vi "MoveHWP primitive v2.vi"(6 "tolerance":sgl, 7 "StopCtrl":bool, 8 "error in (no error)":errorcluster, 9 "DesiredAngle":sgl, 10 "HomeTheStage":bool, 11 "Automation Refnum in":refnum<k7>) -> (0 "error out":errorcluster, 1 "running error out":errorcluster, 2 "GetPosition_Position":sgl, 3 "GetStatusBits_Bits continual":i32 format="%b", 5 "CurrentAngle":sgl)   [LabVIEW 2013]
uses:
  <vilib>/Analysis/1siggen.llb/Ramp Pattern by Delta.vi
  <vilib>/Analysis/NI_AALBase.lvlib
panel:
  out "Array":sgl[](array[numeric])
  out "XY Graph":T1(graph)
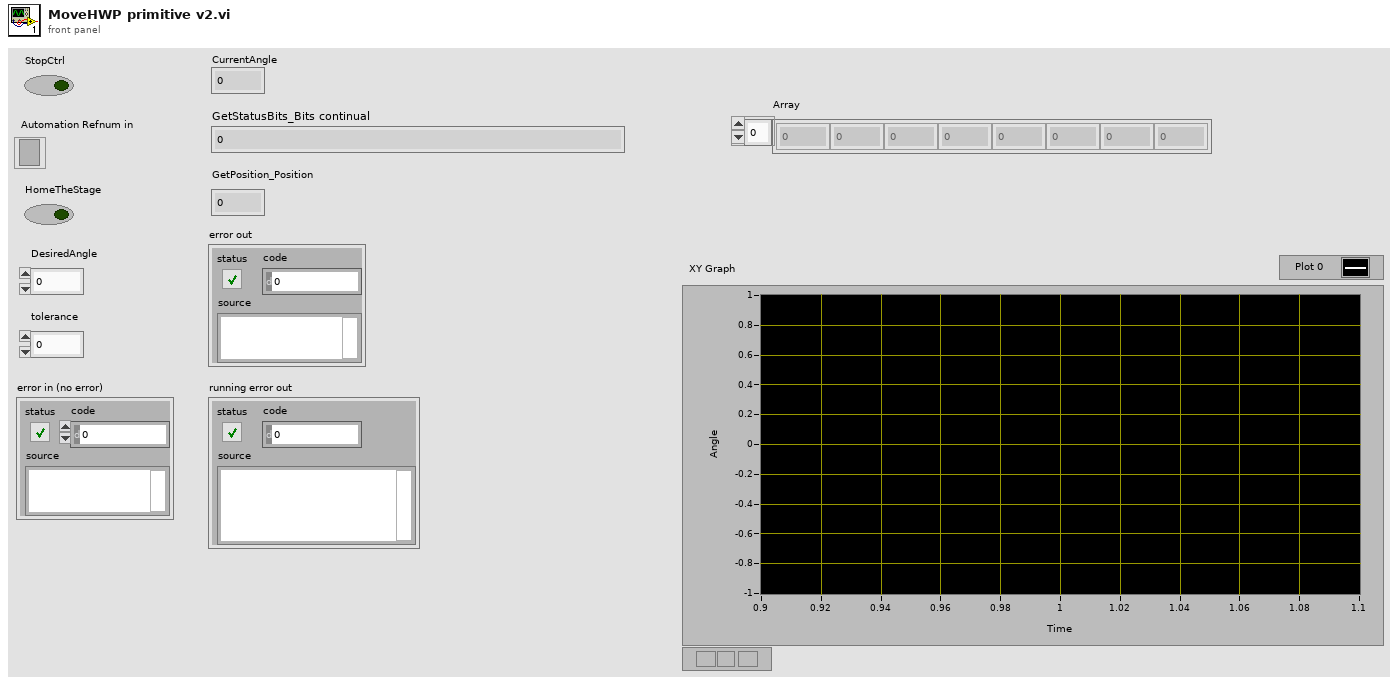
[diagram p1: front panel]
types:
  T1 = cluster{"Ramp Pattern":dbl[], "Array of Continuous Angles":dbl[]}
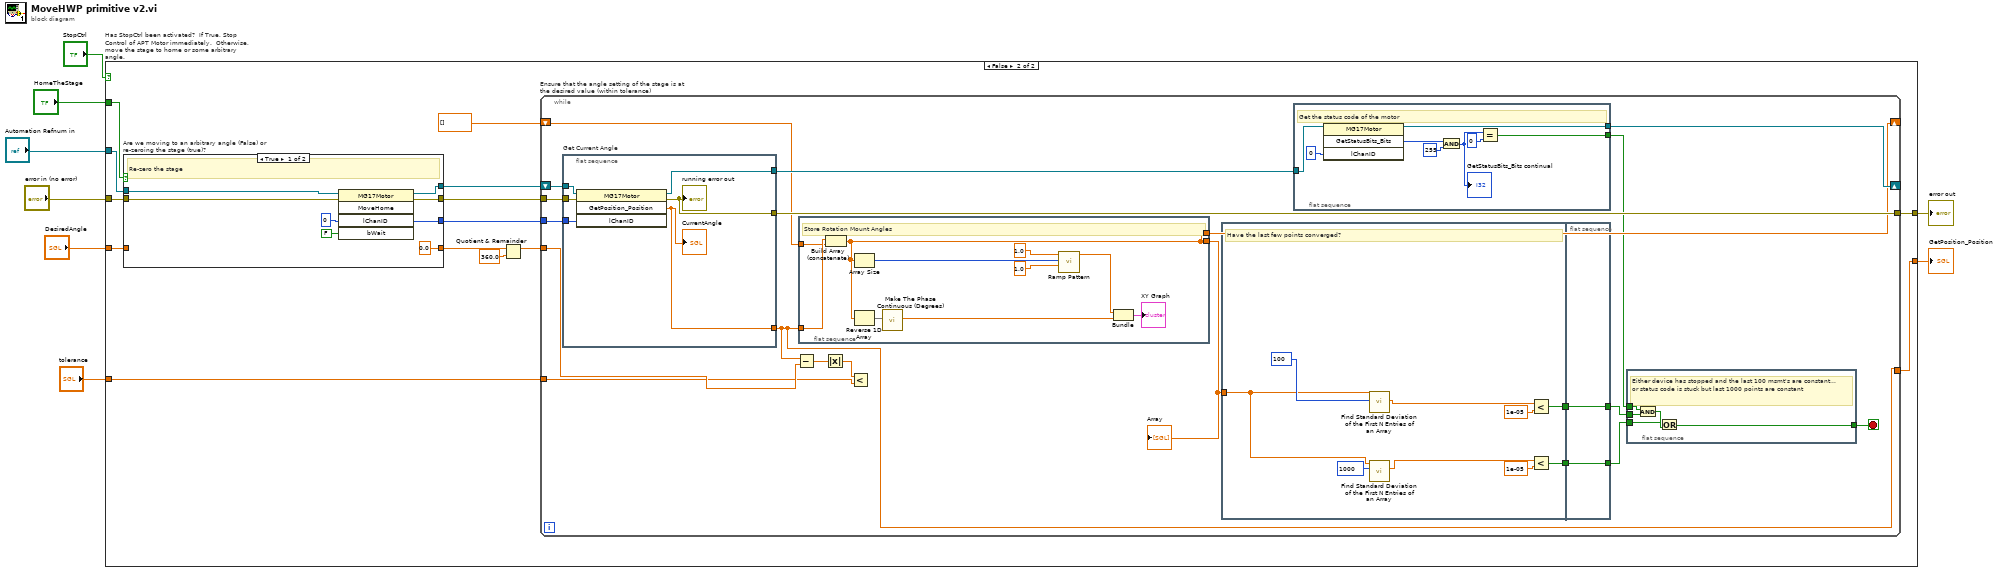
[diagram p0: block diagram]
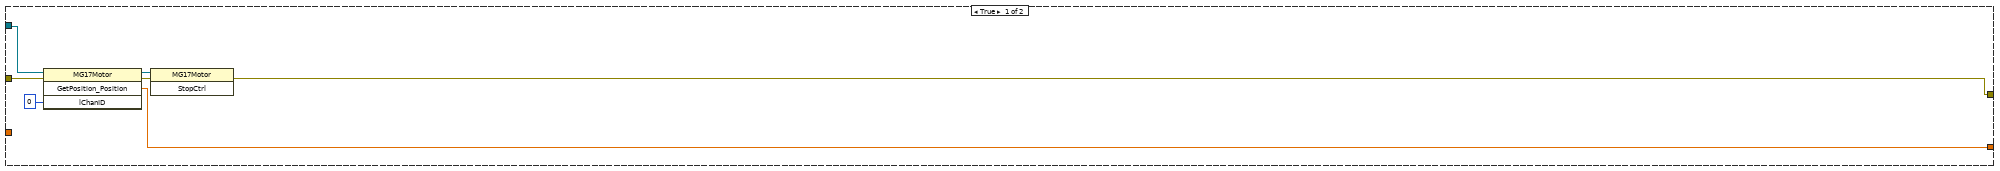
[diagram p2: hidden frame]
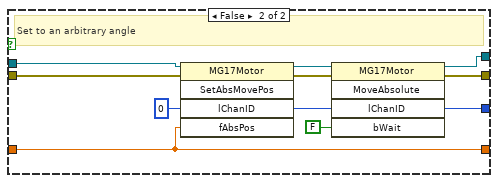
[diagram p3: hidden frame]
diagram:
  n1 = case "Has StopCtrl been activated?  If True, Stop Control of APT Motor immediately.  Otherwise, move the stage to home or some arbitrary angle." shown="False" "StopCtrl" {
    tunnel: "Automation Refnum in" -> [w15 w29]
    tunnel: "error in (no error)" -> [w14 w28]
    tunnel: [w10 w22] -> w3
    tunnel: [w9 w23] -> w2
    tunnel: "HomeTheStage" -> [_ w20]
    tunnel: "DesiredAngle" -> [_ w19]
    tunnel: "tolerance" -> [_ w18]
    frame True {
      n2 = invoke class="MG17Motor" method="GetPosition_Position"(reference=w15, error in=w14, "lChanID"=0) -> (reference out=w12:refnum<k7>, error out=w11:errorcluster, "GetPosition_Position"=w9:sgl)  [unwired: 1 in, 1 out]
      n3 = invoke class="MG17Motor" method="StopCtrl"(reference=w12, error in=w11) -> (error out=w10:errorcluster)  [unwired: 1 in, 2 out]
    }
    frame False {
      n4 = case "Are we moving to an arbitrary angle (False) or re-zeroing the stage (true)?" shown="True" w20 {
        tunnel: w29 -> [w95 w103]
        tunnel: w28 -> [w94 w102]
        tunnel: [w93 w101] -> w27
        tunnel: [sgl 0.0 ("Angle") w98] -> w26
        tunnel: [w91 w99] -> w25
        tunnel: [w90 w100] -> w24
        tunnel: w19 -> [_ w98]
        frame True {
          # "Re-zero the stage"
          n5 = invoke class="MG17Motor" method="MoveHome"(reference=w95, error in=w94, "lChanID"=0, "bWait"=FALSE) -> (reference out=w93:refnum<k7>, error out=w90:errorcluster, "lChanID"=w91:i32)  [unwired: 1 in, 2 out]
        }
        frame False {
          # "Set to an arbitrary angle"
          n6 = invoke class="MG17Motor" method="SetAbsMovePos"(reference=w103, error in=w102, "lChanID"=0, "fAbsPos"=w98) -> (reference out=w108:refnum<k7>, error out=w107:errorcluster, "lChanID"=w106:i32)  [unwired: 1 in, 2 out]
          n7 = invoke class="MG17Motor" method="MoveAbsolute"(reference=w108, error in=w107, "lChanID"=w106, "bWait"=FALSE) -> (reference out=w101:refnum<k7>, error out=w100:errorcluster, "lChanID"=w99:i32)  [unwired: 1 in, 2 out]
        }
      }
      n8 = Quotient & Remainder(x=w26, y=sgl 360.0) -> (x-y*floor(x/y)=w17:sgl)  [unwired: 1 out]
      n9 = while "Ensure that the angle setting of the stage is at the desired value (within tolerance)" {
        tunnel: w25 -> [w49]
        tunnel: w24 -> [w47]
        tunnel: w17 -> [w38]
        tunnel: [w44] -> w22
        tunnel: [w41] -> w23
        shift-right: [w42] -> _
        shift-left: w27 -> [w48]
        shift-right: [w39] -> _
        shift-left: sgl[] [] -> [w40]
        tunnel: w18 -> [w35]
        stop <- w33 stop-if-true
        n10 = flat-sequence "Get Current Angle" {
          tunnel: w49 -> [w79]
          tunnel: w48 -> [w78]
          tunnel: w47 -> [w77]
          tunnel: [w76] -> w44
          tunnel: [w75] -> w43
          tunnel: [w74] -> w41
          frame #0 {
            n11 = invoke class="MG17Motor" method="GetPosition_Position"(reference=w78, error in=w77, "lChanID"=w79) -> (reference out=w75:refnum<k7>, error out=w76:errorcluster, "GetPosition_Position"=w74:sgl)  [unwired: 1 in, 1 out]
            "running error out" <- w76
            "CurrentAngle" <- w74
          }
        }
        n12 = Subtract(x=w41, y=w38) -> (x-y=w46:sgl)
        n13 = flat-sequence {
          tunnel: w41 -> [w89]
          tunnel: w40 -> [w88]
          tunnel: [w80] -> w30
          tunnel: [w80] -> w39
          frame #0 {
            # "Store Rotation Mount Angles"
            n14 = Build Array (concatenate)(w89, w88) -> (w80:sgl[])
            n15 = Array Size(array=w80) -> (size(s)=w85:i32)
            n16 = Reverse 1D Array(array=w80) -> (reversed array=w82:sgl[])
            n17 = call "Make The Phase Continuous (Degrees).vi"("Array of Angles\nDiscontinuous"=w82) -> ("Array of Continuous Angles"=w81:dbl[])  [unwired: 10 in]
            n18 = call-poly <vilib>:"Ramp Pattern.vi"("start"=1.0, "end"=w85, "delta"=1.0) -> ("Ramp Pattern"=w84:dbl[])  [unwired: 6 in, 2 out]
            n19 = Bundle("Ramp Pattern"=w84, "Array of Continuous Angles"=w81) -> (→"XY Graph":T1)  [unwired: 1 in]
          }
        }
        n20 = Absolute Value(x=w46) -> (abs(x)=w45:sgl)
        n21 = Less?(x=w45, y=w35) -> ()  [unwired: 1 out]
        n22 = flat-sequence {
          tunnel: w30 -> [w63]
          tunnel: [w70] -> w34
          tunnel: [w68] -> w32
          tunnel: [w73] -> w36
          tunnel: w34 -> [w73]
          tunnel: [w72] -> w31
          tunnel: w32 -> [w72]
          frame #0 {
            # "Have the last few points converged?"
            n23 = call "Find Standard Deviation of the First N Entries of an Array.vi"("N"=100 ("length"), "Array"=w63) -> ("standard deviation"=w67:dbl)  [unwired: 9 in]
            n24 = call "Find Standard Deviation of the First N Entries of an Array.vi"("N"=u32 1000, "Array"=w63) -> ("standard deviation"=w65:dbl)  [unwired: 9 in]
            n25 = Less?(x=w67, y=1e-05) -> (x < y?=w70:bool)
            n26 = Less?(x=w65, y=1e-05) -> (x < y?=w68:bool)
          }
          frame #1 {
          }
        }
        n27 = flat-sequence {
          tunnel: w43 -> [w61]
          tunnel: [w60] -> w42
          tunnel: [w55] -> w37
          frame #0 {
            # "Get the status code of the motor"
            n28 = invoke class="MG17Motor" method="GetStatusBits_Bits"(reference=w61, "lChanID"=0) -> (reference out=w60:refnum<k7>, "GetStatusBits_Bits"=w59:i32)  [unwired: 2 in, 2 out]
            n29 = And(x=w59, y=255) -> (x .and. y?=w57:i32)
            "GetStatusBits_Bits continual" <- w57
            n30 = Equal?(x=w57, y=0) -> (x = y?=w55:bool)
          }
        }
        n31 = flat-sequence {
          tunnel: w37 -> [w53]
          tunnel: w36 -> [w52]
          tunnel: [w51] -> w33
          tunnel: w31 -> [w50]
          frame #0 {
            # "Either device has stopped and the last 100 msmt's are constant... or status code is stuck but last 1000 points are constant"
            n32 = And(x=w53, y=w52) -> (x .and. y?=w54:bool)
            n33 = Or(x=w50, y=w54) -> (x .or. y?=w51:bool)
          }
        }
        "Array" <- w30
      }
    }
  }
  "error out" <- w3
  "GetPosition_Position" <- w2
